vi "Launch New Chat Window.vi"(8 "error in (no error)":errorcluster, 11 "Server in":refnum<class "Server.lvclass">) -> (0 "error out":errorcluster, 3 "Server out":refnum<class "Server.lvclass">)   [LabVIEW 2020, in "Server.lvlib" / "Server.lvclass"]
uses:
  Server.lvclass
  C:/Program Files/National Instruments/LabVIEW 2020/vi.lib/ActorFramework/Actor/Actor.lvclass
  Chat Window Model/Chat Window Model/Chat Window Model.lvclass
  <vilib>/ActorFramework/Message Enqueuer/Message Enqueuer.lvclass
  Chat Window Model/Chat Window Model/Chat Window Model.lvclass/Chat Window Model.ctl
  <vilib>/ActorFramework/Actor/Actor.lvclass/Actor.ctl
  <vilib>/ActorFramework/Message Enqueuer/Message Enqueuer.lvclass/Message Enqueuer.ctl
  Server.lvclass/Server.ctl
  Server Messages/Enable Controls Msg/Enable Controls Msg.lvclass/Enable Controls Msg.ctl
  Chat Window Model/Chat Window Model Messages/Update Status Log Msg/Update Status Log Msg.lvclass/Update Status Log Msg.ctl
  Chat Window Model/Chat Window Model Messages/Update Online List Msg/Update Online List Msg.lvclass/Update Online List Msg.ctl
  <vilib>/ActorFramework/Message Enqueuer/Init from Existing Queue.vi
  <vilib>/ActorFramework/Message Enqueuer/Enqueue.vi
  Server Messages/Enable Controls Msg/Enable Controls Msg.lvclass
  C:/Program Files/National Instruments/LabVIEW 2020/vi.lib/ActorFramework/Message/Message.lvclass
  Chat Window Model/Chat Window Model Messages/Update Status Log Msg/Update Status Log Msg.lvclass
  Chat Window Model/Chat Window Model Messages/Update Online List Msg/Update Online List Msg.lvclass
  <vilib>/ActorFramework/Message Priority Queue/Priority Enqueue.vi
  <vilib>/ActorFramework/Actor/Actor.lvclass
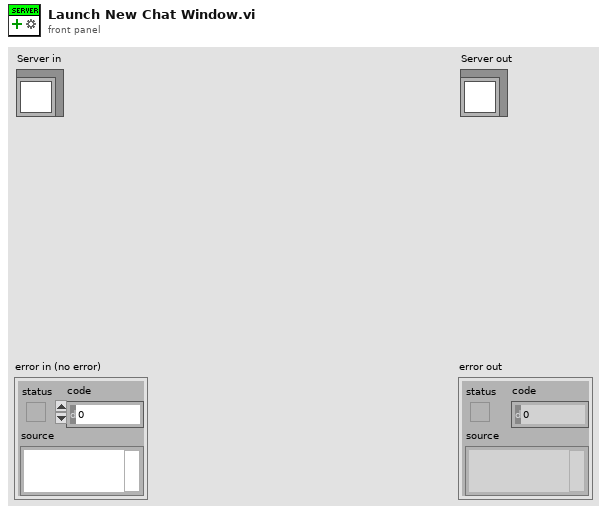
[diagram p1: front panel]
types:
  T1 = cluster{"Enqueuer":refnum<class "Message Enqueuer.lvclass">, "Status":string}
  T2 = enum8{"Enabled", "Disabled", "Disabled and Grayed Out"}
  T3 = map{string, cluster{"Enqueuer":refnum<class "Message Enqueuer.lvclass">, "Status":string}}
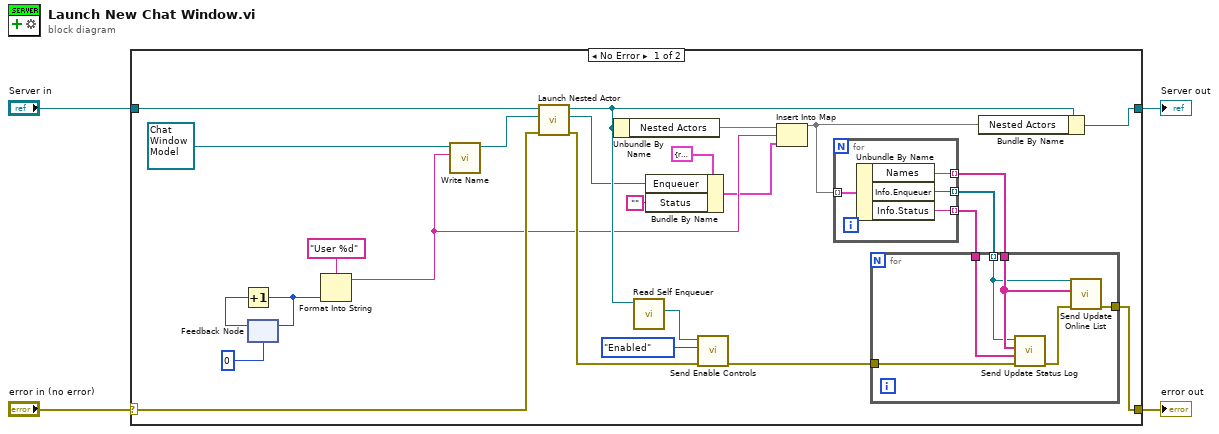
[diagram p0: block diagram]
diagram:
  n1 = case shown="No Error" "error in (no error)" {
    selector: "error in (no error)" -> [w28 w41]
    tunnel: [w20 w41] -> w3
    tunnel: [w21 w40] -> w1
    tunnel: "Server in" -> [w29 w40]
    frame No Error {
      n2 = feedback #1(0) -> (w25:i32)
      n3 = Increment(x=w25) -> (x+1=w23:i32)
      n4 = feedback-in #1(w23) -> ()
      n5 = Format Into String(format string="User %d", w23) -> (resulting string=w13:string)  [unwired: 2 in, 1 out]
      n6 = call "Write Name.vi"("Name"=w13, "Chat Window Model in"=refnum<class "Chat Window Model.lvclass"> refnum ("Chat Window Model.lvlib:Chat Window Model.lvclass")) -> ("Chat Window Model out"=w27:refnum<class "Chat Window Model.lvclass">)  [unwired: 8 in, 1 out]
      n7 = call <vilib>:"Launch Nested Actor.vi"("error in (no error)"=w28, "Nested Actor"=w27, "Caller Actor in"=w29) -> ("error out"=w18:errorcluster, "Nested Actor's Enqueuer"=w11:refnum<class "Message Enqueuer.lvclass">, "Caller Actor out"=w17:refnum<class "Server.lvclass">)  [unwired: 6 in]
      n8 = Unbundle By Name(w17) -> ("Nested Actors"=w14:T3)
      n9 = call <vilib>:"Read Self Enqueuer.vi"("Actor"=w17) -> ("Self Enqueuer"=w16:refnum<class "Message Enqueuer.lvclass">)  [unwired: 10 in]
      n10 = Bundle By Name(cluster=T1 {"Enqueuer"=refnum, "Status"=""} ("value"), "Enqueuer"=w11, "Status"="") -> (w9:T1)
      n11 = call "Send Enable Controls.vi"("error in (no error)"=w18, "Disabled"=T2."Enabled", "Message Enqueuer"=w16) -> ("error out"=w19:errorcluster)  [unwired: 7 in, 1 out]
      n12 = Insert Into Map(map in=w14, key=w13, value=w9) -> (map out=w8:T3)  [unwired: 2 out]
      n13 = for {
        tunnel: [w32] -> w7 mode=indexing
        tunnel: w8 -> [w33] mode=indexing
        tunnel: [w31] -> w6 mode=indexing
        tunnel: [w30] -> w5 mode=indexing
        n14 = Unbundle By Name(w33) -> ("Names"=w32:string, "Info.Enqueuer"=w31:refnum<class "Message Enqueuer.lvclass">, "Info.Status"=w30:string)
      }
      n15 = for {
        tunnel: [w38] -> w20
        tunnel: w19 -> [w37]
        tunnel: w7 -> [w36]
        tunnel: w6 -> [w35] mode=indexing
        tunnel: w5 -> [w34]
        n16 = call "Send Update Status Log.vi"("error in (no error)"=w37, "Status List"=w34, "Names"=w36, "Message Enqueuer"=w35) -> ("error out"=w39:errorcluster)  [unwired: 6 in, 1 out]
        n17 = call "Send Update Online List.vi"("error in (no error)"=w39, "Online Users"=w36, "Message Enqueuer"=w35) -> ("error out"=w38:errorcluster)  [unwired: 7 in, 1 out]
      }
      n18 = Bundle By Name(cluster=w17, "Nested Actors"=w8) -> (w21:refnum<class "Server.lvclass">)
    }
    frame Error {
    }
  }
  "error out" <- w3
  "Server out" <- w1
